vi "createSocket.vi"() -> (1 "error out":errorcluster, 2 "socket out":refnum<class "zmq_socket.lvclass">, 3 "context out":refnum<class "zmq_context.lvclass">)   [LabVIEW 2020]
uses:
  <vilib>/addons/zeromq/zmq_socket.lvclass
  <vilib>/addons/zeromq/zmq_context.lvclass
  <vilib>/addons/zeromq/socket_type.ctl
  <vilib>/addons/zeromq/zeromq.lvlib
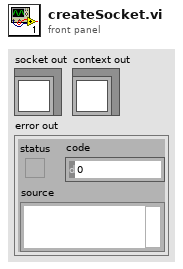
[diagram p1: front panel]
types:
  T1 = typedef "zeromq.lvlib/socket_type.ctl" = enum8{"ZMQ_PAIR", "ZMQ_PUB", "ZMQ_SUB", "ZMQ_REQ", "ZMQ_REP", "ZMQ_DEALER", "ZMQ_ROUTER", "ZMQ_PULL", "ZMQ_PUSH", "ZMQ_XPUB", "ZMQ_XSUB", "ZMQ_STREAM", "ZMQ_SERVER", "ZMQ_CLIENT", "ZMQ_RADIO", "ZMQ_DISH", "ZMQ_GATHER", "ZMQ_SCATTER", "ZMQ_DGRAM"}
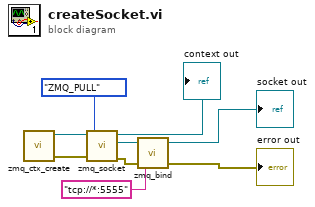
[diagram p0: block diagram]
diagram:
  n1 = call <vilib>:"zmq_ctx_create.vi"() -> ("error out"=w6:errorcluster, "context out"=w9:refnum<class "zmq_context.lvclass">)  [unwired: 4 in]
  n2 = call <vilib>:"zmq_socket.vi"("error in"=w6, "socket type"=socket_type."ZMQ_PULL", "context in"=w9) -> ("error out"=w5:errorcluster, "socket out"=w8:refnum<class "zmq_socket.lvclass">, "context out"=→"context out":refnum<class "zmq_context.lvclass">)  [unwired: 2 in]
  n3 = call <vilib>:"zmq_bind.vi"("error in"=w5, "endpoint"="tcp://*:5555", "socket in"=w8) -> ("error out"=→"error out":errorcluster, "socket out"=→"socket out":refnum<class "zmq_socket.lvclass">)  [unwired: 1 in]
